vi "Debugger.vi"(8 "error in (no error)":errorcluster, 11 "Debugger In":refnum<class "Debugger.lvclass">) -> (0 "error out":errorcluster, 3 "Debugger Out":refnum<class "Debugger.lvclass">)   [LabVIEW 2020, in "Debugger.lvclass"]
uses:
  Debugger.lvclass
  Chronological List/Chronological List.lvclass
  C:/Users/anton/Documents/GitHub/triarc-debugger/source/Debug Log View/Debug Log View.lvclass
  Debugger.lvclass/Debugger.ctl
  Debug Log View/Debug Log View.lvclass
  TypeDefs/Debug Data.ctl
  <vilib>/Utility/miscctls.llb/LVPositionTypeDef.ctl
  <vilib>/Utility/miscctls.llb/LVRowAndColumnTypeDef.ctl
panel:
  in  "Processes":i32[](listbox)
  in  "Messages":i32[](listbox)
  in  "Message Log":i32(listbox)
  in  "Clear":bool
  out "Message data":variant
  in  "Received Messages":bool=TRUE
  in  "Sent Messages":bool=TRUE
  in  "Auto-Scroll":bool=TRUE
  in  "View":enum32{"Chronological", "Grouped"}(radio)
  out "Debugger enabled?":bool
  # "- Grouping"
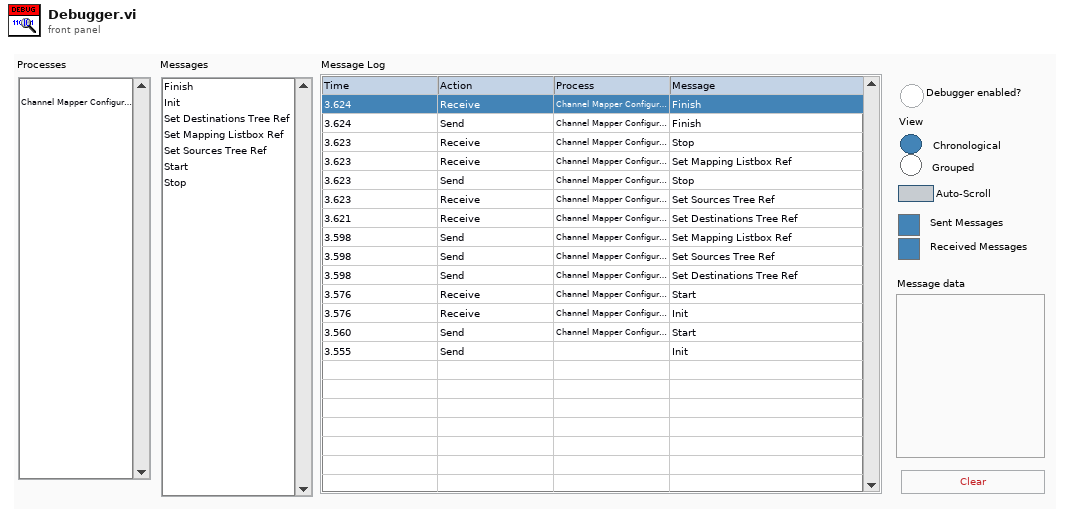
[diagram p1: front panel]
types:
  T1 = cluster{"Action":string, "Call Chain":string, "Process":string, "Message":string, "Message Data":variant, "Time":u32}
  T2 = typedef "Debugger.lvclass/Debug Data.ctl" = cluster{"Action":string, "Call Chain":string, "Process":string, "Message":string, "Message Data":variant, "Time":u32}
  T3 = typedef "LVPositionTypeDef.ctl" = cluster{"Left":i32, "Top":i32}
  T4 = typedef "LVRowAndColumnTypeDef.ctl" = cluster{"Row":i32, "Column":i32}
  T5 = typedef "LVRectTypeDef.ctl" = cluster{"Left":i16, "Top":i16, "Right":i16, "Bottom":i16}
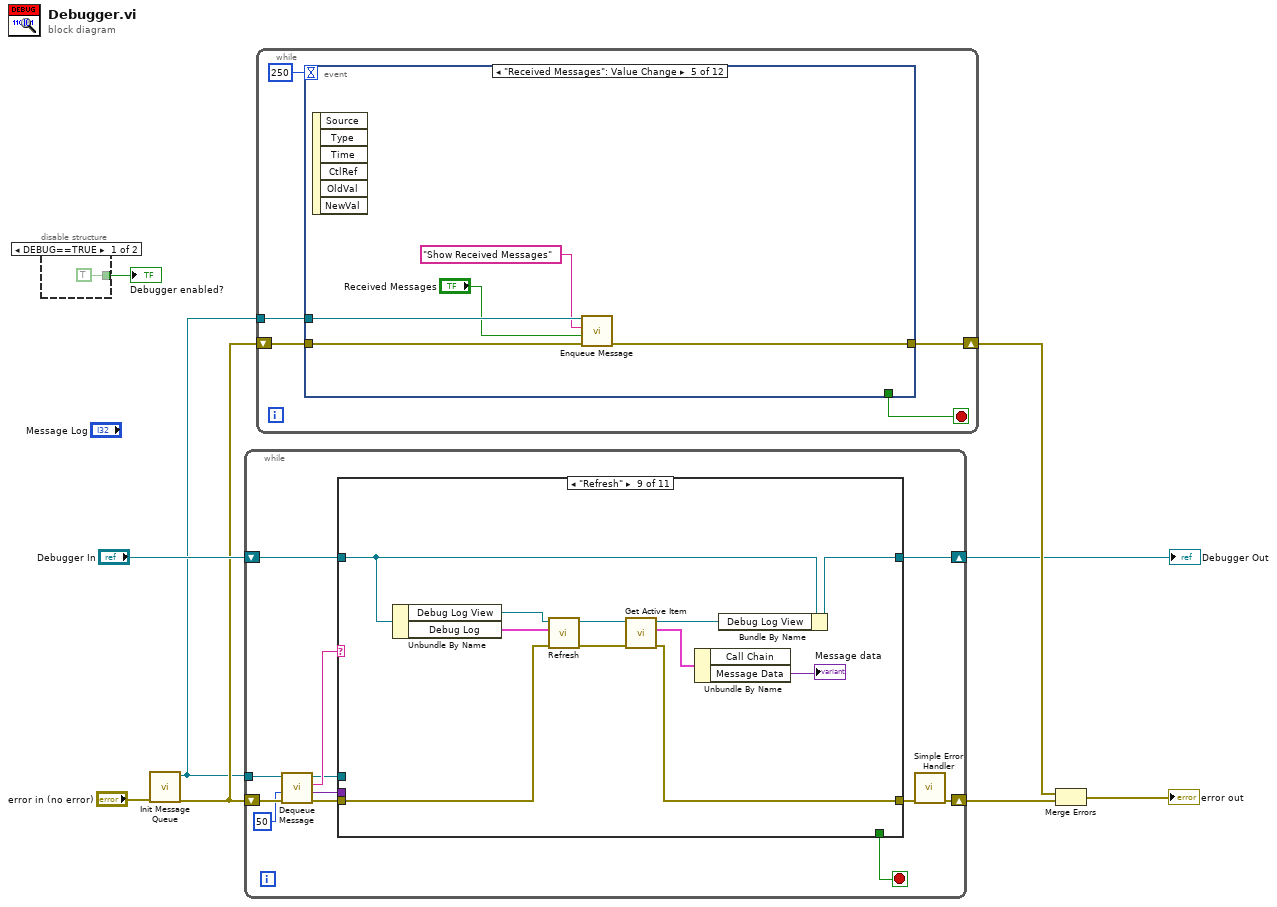
[diagram p0: block diagram]
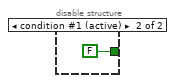
[diagram p2: hidden frame]
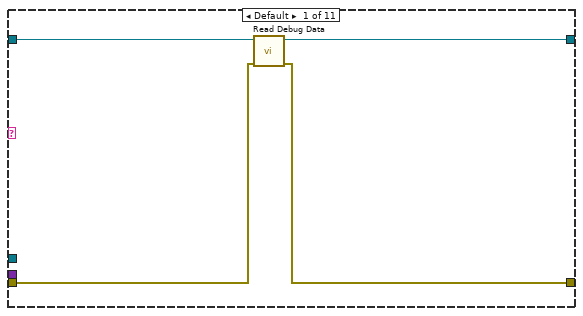
[diagram p3: hidden frame]
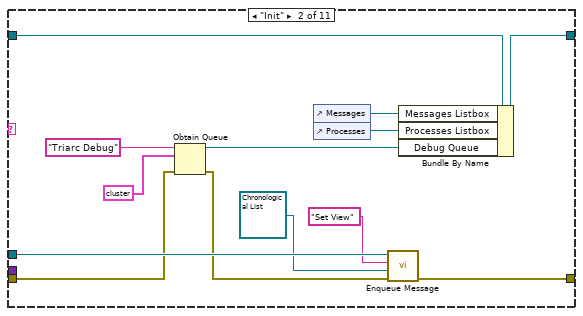
[diagram p4: hidden frame]
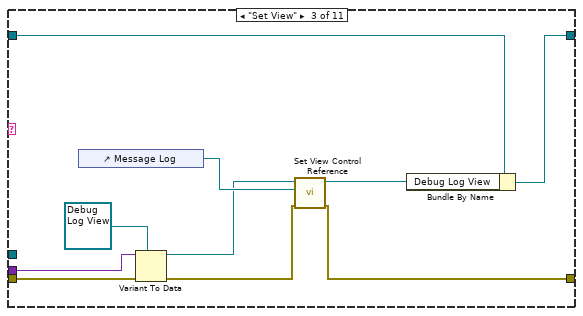
[diagram p5: hidden frame]
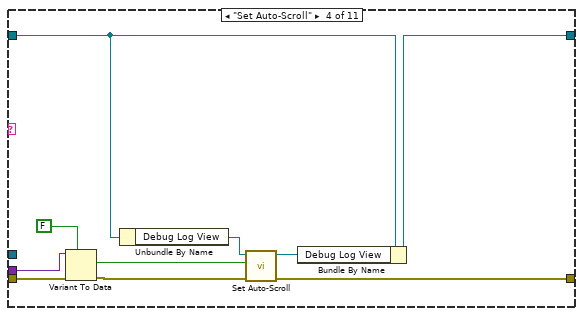
[diagram p6: hidden frame]
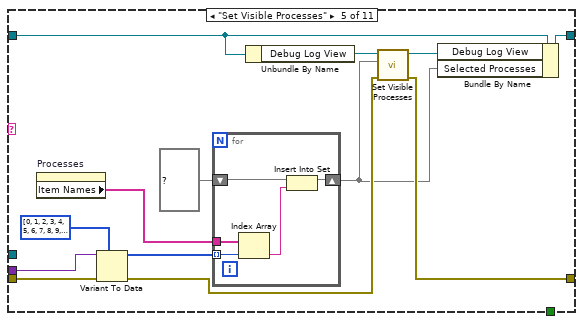
[diagram p7: hidden frame]
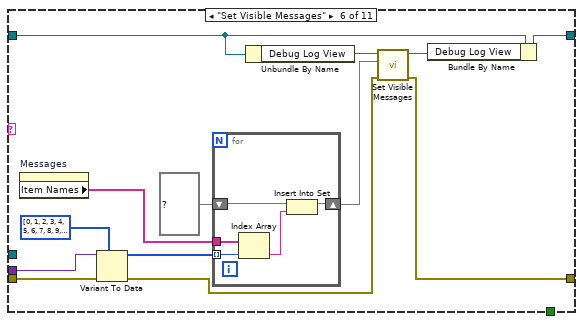
[diagram p8: hidden frame]
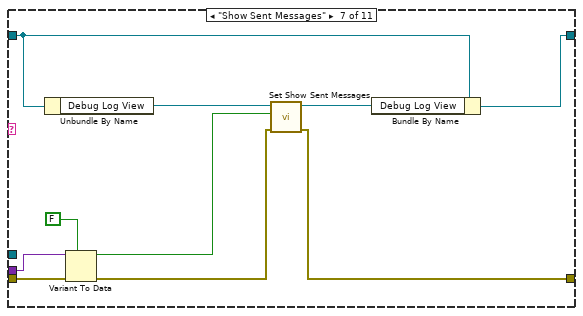
[diagram p9: hidden frame]
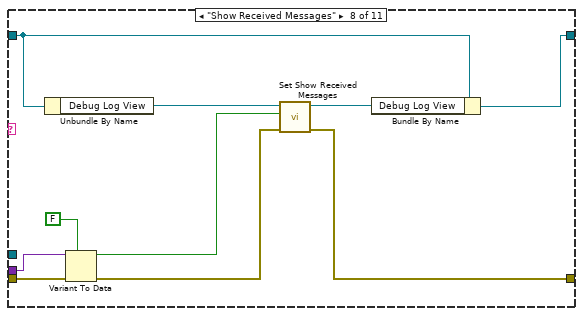
[diagram p10: hidden frame]
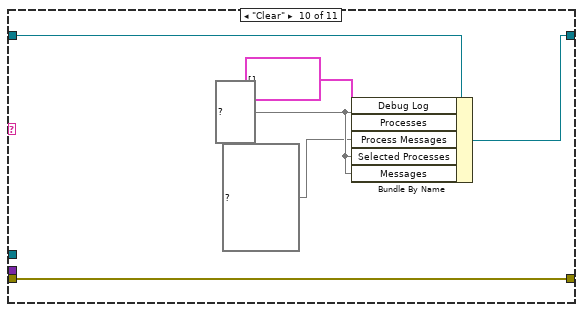
[diagram p11: hidden frame]
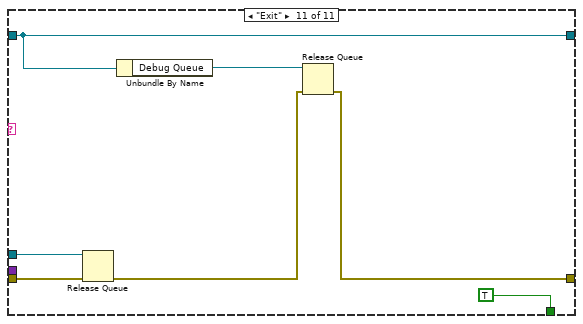
[diagram p12: hidden frame]
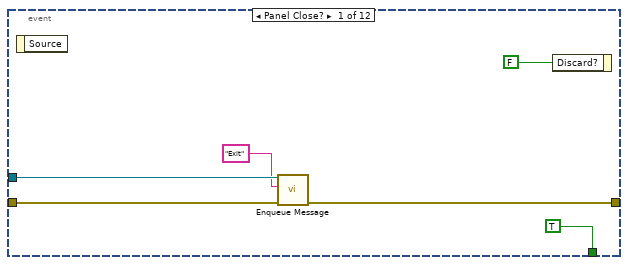
[diagram p13: hidden frame]
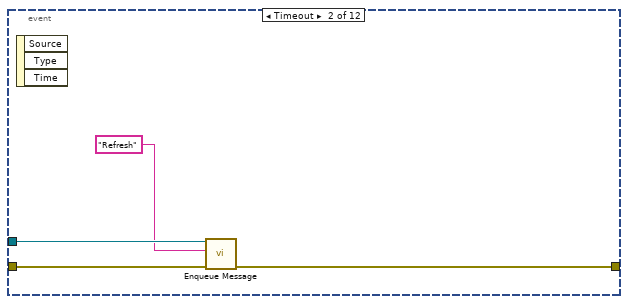
[diagram p14: hidden frame]
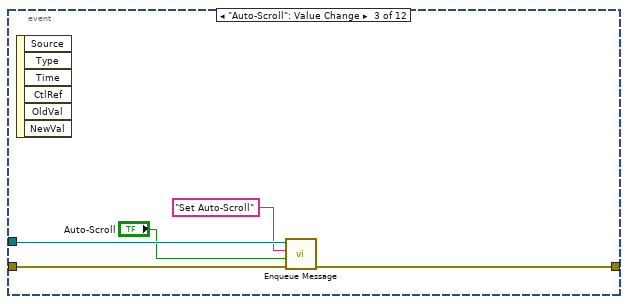
[diagram p15: hidden frame]
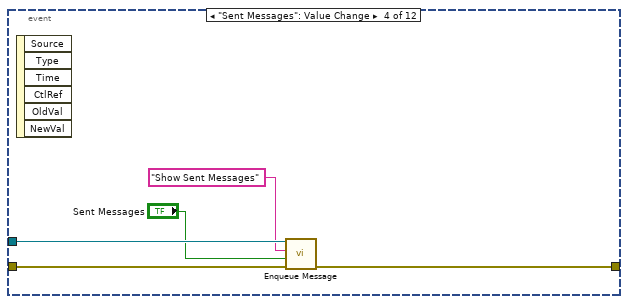
[diagram p16: hidden frame]
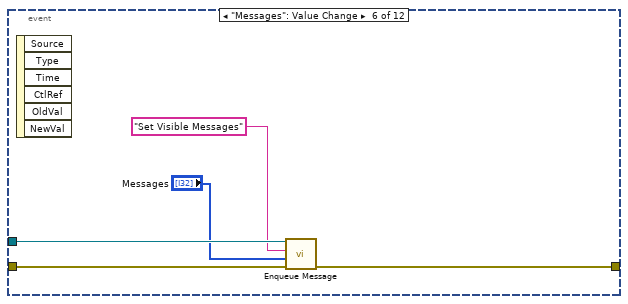
[diagram p17: hidden frame]
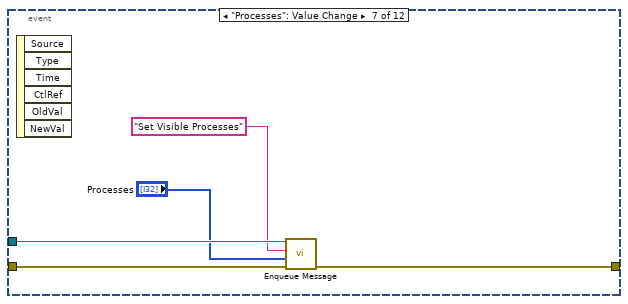
[diagram p18: hidden frame]
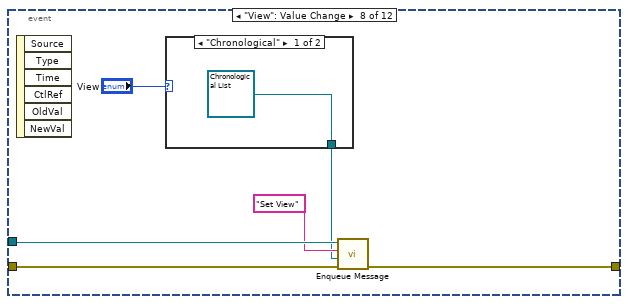
[diagram p19: hidden frame]
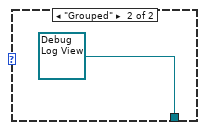
[diagram p20: hidden frame]
diagram:
  n1 = disable-structure shown="DEBUG==TRUE" {
    disable-tunnel: [TRUE FALSE ("Debugger enabled?")] -> w8
    frame condition #0 {
    }
    frame condition #1 (active) {
    }
  }
  "Debugger enabled?" <- w8
  n2 = call "Init Message Queue.vi"("error in (no error)"="error in (no error)") -> ("error out"=w5:errorcluster, "Queue out"=w4:refnum<queue>)  [unwired: 9 in]
  n3 = while {
    shift-right: [w22] -> w3
    shift-left: "Debugger In" -> [w23]
    shift-right: [w12] -> w1
    shift-left: w5 -> [w18]
    tunnel: w4 -> [w21]
    stop <- w14 stop-if-true
    n4 = call "Dequeue Message.vi"("error in (no error)"=w18, "timeout in ms (-1)"=50, "Queue in"=w21) -> ("error out"=w16:errorcluster, "Message Data"=w19:variant, "Message"=w20:string, "Queue out"=w15:refnum<queue>)  [unwired: 5 in]
    n5 = case shown="\"Refresh\"" w20 {
      tunnel: [w24 w36 w48 w52 w66 w82 w102 w112 w125 w132 w138] -> w22
      tunnel: w23 -> [w27 w40 w49 w53 w67 w83 w103 w113 w127 w133 w138]
      tunnel: w19 -> [_ _ w43 w59 w73 w91 w105 w115 _ _ _]
      tunnel: [w25 w32 w46 w55 w64 w80 w97 w107 w119 w131 w137] -> w17
      tunnel: w16 -> [w26 w34 w45 w60 w72 w90 w106 w116 w126 w131 w135]
      tunnel: w15 -> [_ w39 _ _ _ _ _ _ _ _ w136]
      tunnel: [_ _ _ _ _ _ _ _ _ _ TRUE] -> w14
      frame Default {
        n6 = call "Read Debug Data.vi"("error in (no error)"=w26, "Debugger in"=w27) -> ("error out"=w25:errorcluster, "Debugger out"=w24:refnum<class "Debugger.lvclass">)  [unwired: 8 in]
      }
      frame "Init" {
        n7 = Obtain Queue(name (unnamed)="Triarc Debug", element data type=T1 {"Action"="", "Call Chain"="", "Process"="", "Message"="", "Message Data"=variant, "Time"=0} ("output cluster"), error in (no error)=w34) -> (queue out=w35:refnum<queue>, error out=w33:errorcluster)  [unwired: 2 in, 1 out]
        n8 = control-ref of="Messages"() -> (w28:refnum<vi>)
        n9 = control-ref of="Processes"() -> (w29:refnum<vi>)
        n10 = call "Enqueue Message.vi"("error in (no error)"=w33, "Message Data"=refnum<class "Chronological List.lvclass"> refnum ("Debugger.lvlib:Chronological List.lvclass"), "Message"="Set View", "Queue in"=w39) -> ("error out"=w32:errorcluster)  [unwired: 6 in, 1 out]
        n11 = Bundle By Name(cluster=w40, "Messages Listbox"=w28, "Processes Listbox"=w29, "Debug Queue"=w35) -> (w36:refnum<class "Debugger.lvclass">)
      }
      frame "Set View" {
        n12 = control-ref of="Message Log"() -> (w50:refnum<vi>)
        n13 = Variant To Data(error in=w45, type=refnum<class "Debug Log View.lvclass"> refnum ("Debug Log View"), Variant=w43) -> (data=w41:refnum<class "Debug Log View.lvclass">, error out=w44:errorcluster)
        n14 = call-dynamic "Set View Control Reference.vi"("error in (no error)"=w44, "View Control"=w50, "Debug Log View in"=w41) -> ("error out"=w46:errorcluster, "Debug Log View out"=w47:refnum<class "Debug Log View.lvclass">)  [unwired: 7 in]
        n15 = Bundle By Name(cluster=w49, "Debug Log View"=w47) -> (w48:refnum<class "Debugger.lvclass">)
      }
      frame "Set Auto-Scroll" {
        n16 = Variant To Data(error in=w60, type=FALSE, Variant=w59) -> (data=w57:bool, error out=w56:errorcluster)
        n17 = Unbundle By Name(w53) -> ("Debug Log View"=w54:refnum<class "Debug Log View.lvclass">)
        n18 = call-dynamic "Set Auto-Scroll.vi"("error in (no error)"=w56, "Auto-Scroll?"=w57, "Debug Log View in"=w54) -> ("error out"=w55:errorcluster, "Debug Log View out"=w51:refnum<class "Debug Log View.lvclass">)  [unwired: 7 in]
        n19 = Bundle By Name(cluster=w53, "Debug Log View"=w51) -> (w52:refnum<class "Debugger.lvclass">)
      }
      frame "Set Visible Processes" {
        n20 = property on="Processes" class="LstBox (strict)"() -> ("Item Names"=w62:string[])  [unwired: 2 in, 2 out]
        n21 = Variant To Data(error in=w72, type=i32[] [0, 1, 2, 3, 4, 5, 6, 7, 8, 9, 10, 11, 12, 13, 14, 15, 16, 17, 18, 19, 20, 21, 22] ("Message Filter"), Variant=w73) -> (data=w70:i32[], error out=w63:errorcluster)
        n22 = for {
          tunnel: w62 -> [w78]
          tunnel: w70 -> [w77] mode=indexing
          shift-right: [w74] -> w61
          shift-left: set{string} {} ("set in") -> [w76]
          n23 = Index Array(array=w78, index=w77) -> (element=w75:string)
          n24 = Insert Into Set(10:w75, 11:w76) -> (3:w74:set{string})  [unwired: 1 out]
        }
        n25 = Unbundle By Name(w67) -> ("Debug Log View"=w68:refnum<class "Debug Log View.lvclass">)
        n26 = call-dynamic "Set Visible Processes.vi"("error in (no error)"=w63, "Processes"=w61, "Debug Log View In"=w68) -> ("error out"=w64:errorcluster, "Debug Log View Out"=w65:refnum<class "Debug Log View.lvclass">)  [unwired: 7 in]
        n27 = Bundle By Name(cluster=w67, "Debug Log View"=w65, "Selected Processes"=w61) -> (w66:refnum<class "Debugger.lvclass">)
      }
      frame "Set Visible Messages" {
        n28 = property on="Messages" class="LstBox (strict)"() -> ("Item Names"=w88:string[])  [unwired: 2 in, 2 out]
        n29 = Variant To Data(error in=w90, type=i32[] [0, 1, 2, 3, 4, 5, 6, 7, 8, 9, 10, 11, 12, 13, 14, 15, 16, 17, 18, 19, 20, 21, 22] ("Message Filter"), Variant=w91) -> (data=w87:i32[], error out=w79:errorcluster)
        n30 = for {
          tunnel: w88 -> [w96]
          tunnel: w87 -> [w95] mode=indexing
          shift-right: [w92] -> w85
          shift-left: set{string} {} ("set in") -> [w94]
          n31 = Index Array(array=w96, index=w95) -> (element=w93:string)
          n32 = Insert Into Set(10:w93, 11:w94) -> (3:w92:set{string})  [unwired: 1 out]
        }
        n33 = Unbundle By Name(w83) -> ("Debug Log View"=w84:refnum<class "Debug Log View.lvclass">)
        n34 = call-dynamic "Set Visible Messages.vi"("error in (no error)"=w79, "Messages"=w85, "Debug Log View in"=w84) -> ("error out"=w80:errorcluster, "Debug Log View out"=w81:refnum<class "Debug Log View.lvclass">)  [unwired: 7 in]
        n35 = Bundle By Name(cluster=w83, "Debug Log View"=w81) -> (w82:refnum<class "Debugger.lvclass">)
      }
      frame "Show Sent Messages" {
        n36 = Unbundle By Name(w103) -> ("Debug Log View"=w99:refnum<class "Debug Log View.lvclass">)
        n37 = Variant To Data(error in=w106, type=FALSE, Variant=w105) -> (data=w100:bool, error out=w101:errorcluster)
        n38 = call-dynamic "Set Show Sent Messages.vi"("error in (no error)"=w101, "Show Sent Messages?"=w100, "Debug Log View In"=w99) -> ("error out"=w97:errorcluster, "Debug Log View Out"=w98:refnum<class "Debug Log View.lvclass">)  [unwired: 7 in]
        n39 = Bundle By Name(cluster=w103, "Debug Log View"=w98) -> (w102:refnum<class "Debugger.lvclass">)
      }
      frame "Show Received Messages" {
        n40 = Unbundle By Name(w113) -> ("Debug Log View"=w109:refnum<class "Debug Log View.lvclass">)
        n41 = Variant To Data(error in=w116, type=FALSE, Variant=w115) -> (data=w110:bool, error out=w111:errorcluster)
        n42 = call-dynamic "Set Show Received Messages.vi"("error in (no error)"=w111, "Show Received Messages?"=w110, "Debug Log View In"=w109) -> ("error out"=w107:errorcluster, "Debug Log View Out"=w108:refnum<class "Debug Log View.lvclass">)  [unwired: 7 in]
        n43 = Bundle By Name(cluster=w113, "Debug Log View"=w108) -> (w112:refnum<class "Debugger.lvclass">)
      }
      frame "Refresh" {
        n44 = Unbundle By Name(w127) -> ("Debug Log View"=w124:refnum<class "Debug Log View.lvclass">, "Debug Log"=w123:T2[])
        n45 = call-dynamic "Refresh.vi"("error in (no error)"=w126, "Debug Log"=w123, "Debug Log View In"=w124) -> ("error out"=w120:errorcluster, "Debug Log View Out"=w122:refnum<class "Debug Log View.lvclass">)  [unwired: 7 in]
        n46 = call-dynamic "Get Active Item.vi"("error in (no error)"=w120, "Debug Log View In"=w122) -> ("error out"=w119:errorcluster, "Debug Data"=w118:T2, "Debug Log View Out"=w121:refnum<class "Debug Log View.lvclass">)  [unwired: 7 in]
        n47 = Unbundle By Name(w118) -> ("Message Data"=→"Message data":variant)  [unwired: 1 out]
        n48 = Bundle By Name(cluster=w127, "Debug Log View"=w121) -> (w125:refnum<class "Debugger.lvclass">)
      }
      frame "Clear" {
        w129 = set{string} {} ("Processes")
        n49 = Bundle By Name(cluster=w133, "Debug Log"=T2[] [], "Processes"=w129, "Process Messages"=map{string, set{string}} {}, "Selected Processes"=w129, "Messages"=w129) -> (w132:refnum<class "Debugger.lvclass">)
      }
      frame "Exit" {
        n50 = Release Queue(queue=w136, error in (no error)=w135) -> (error out=w134:errorcluster)  [unwired: 1 in, 2 out]
        n51 = Unbundle By Name(w138) -> ("Debug Queue"=w139:refnum<queue>)
        n52 = Release Queue(queue=w139, error in (no error)=w134) -> (error out=w137:errorcluster)  [unwired: 1 in, 2 out]
      }
    }
    n53 = call <vilib>:"Simple Error Handler.vi"("error in (no error)"=w17) -> ("error out"=w12:errorcluster)  [unwired: 4 in, 4 out]
  }
  "Debugger Out" <- w3
  n54 = while {
    shift-right: [w145] -> w9
    shift-left: w5 -> [w144]
    tunnel: w4 -> [w141]
    stop <- w143 stop-if-true
    n55 = event shown="[4] \"Received Messages\": Value Change" {
      selector: _ -> [_ _ _ _ _ _ _ _ _ _ _ _]
      dyn-events: _ -> [_ _ _ _ _ _ _ _ _ _ _ _]
      timeout: 250 -> [_ _ _ _ _ _ _ _ _ _ _ _]
      tunnel: [w148 w154 w159 w164 w169 w174 w179 w185 w190 w192 w199 w213] -> w145
      tunnel: w144 -> [w151 w155 w160 w165 w170 w175 w180 w186 w190 w192 w199 w214]
      tunnel: [TRUE _ _ _ _ _ _ _ _ _ _ _] -> w143
      tunnel: w141 -> [w147 w153 w158 w163 w168 w173 w178 w184 _ _ _ w212]
      event Panel Close? {
        n56 = event-data() -> ()  [unwired: 1 in, 1 out]
        n57 = call "Enqueue Message.vi"("error in (no error)"=w151, "Message"="Exit", "Queue in"=w147) -> ("error out"=w148:errorcluster)  [unwired: 7 in, 1 out]
        n58 = event-data("Discard?"=FALSE) -> ()  [unwired: 1 in, 1 out]
      }
      event Timeout {
        n59 = event-data() -> ()  [unwired: 1 in, 3 out]
        n60 = call "Enqueue Message.vi"("error in (no error)"=w155, "Message"="Refresh", "Queue in"=w153) -> ("error out"=w154:errorcluster)  [unwired: 7 in, 1 out]
      }
      event "Auto-Scroll": Value Change {
        n61 = event-data() -> ()  [unwired: 1 in, 6 out]
        n62 = call "Enqueue Message.vi"("error in (no error)"=w160, "Message Data"="Auto-Scroll", "Message"="Set Auto-Scroll", "Queue in"=w158) -> ("error out"=w159:errorcluster)  [unwired: 6 in, 1 out]
      }
      event "Sent Messages": Value Change {
        n63 = event-data() -> ()  [unwired: 1 in, 6 out]
        n64 = call "Enqueue Message.vi"("error in (no error)"=w165, "Message Data"="Sent Messages", "Message"="Show Sent Messages", "Queue in"=w163) -> ("error out"=w164:errorcluster)  [unwired: 6 in, 1 out]
      }
      event "Received Messages": Value Change {
        n65 = event-data() -> ()  [unwired: 1 in, 6 out]
        n66 = call "Enqueue Message.vi"("error in (no error)"=w170, "Message Data"="Received Messages", "Message"="Show Received Messages", "Queue in"=w168) -> ("error out"=w169:errorcluster)  [unwired: 6 in, 1 out]
      }
      event "Messages": Value Change {
        n67 = event-data() -> ()  [unwired: 1 in, 6 out]
        n68 = call "Enqueue Message.vi"("error in (no error)"=w175, "Message Data"="Messages", "Message"="Set Visible Messages", "Queue in"=w173) -> ("error out"=w174:errorcluster)  [unwired: 6 in, 1 out]
      }
      event "Processes": Value Change {
        n69 = event-data() -> ()  [unwired: 1 in, 6 out]
        n70 = call "Enqueue Message.vi"("error in (no error)"=w180, "Message Data"="Processes", "Message"="Set Visible Processes", "Queue in"=w178) -> ("error out"=w179:errorcluster)  [unwired: 6 in, 1 out]
      }
      event "View": Value Change {
        n71 = event-data() -> ()  [unwired: 1 in, 6 out]
        n72 = case shown="\"Chronological\"" "View" {
          tunnel: [refnum<class "Chronological List.lvclass"> refnum ("Debugger.lvlib:Chronological List.lvclass") refnum<class "Debug Log View.lvclass"> refnum ("Debugger.lvlib:Debug Log View.lvclass")] -> w181
          frame "Chronological" {
          }
          frame "Grouped" {
          }
        }
        n73 = call "Enqueue Message.vi"("error in (no error)"=w186, "Message Data"=w181, "Message"="Set View", "Queue in"=w184) -> ("error out"=w185:errorcluster)  [unwired: 6 in, 1 out]
      }
      event Pane Size {
        n74 = event-data() -> ()  [unwired: 1 in, 1 out]
        n75 = property on="Processes" class="LstBox (strict)"("Position"=T3 {"Left"=2, "Top"=2}) -> ()  [unwired: 2 in, 2 out]
      }
      event Pane Size {
        n76 = event-data() -> ()  [unwired: 1 in, 6 out]
        n77 = property on="Messages" class="LstBox (strict)"("Position"=T3 {"Left"=2, "Top"=2}) -> ()  [unwired: 2 in, 2 out]
      }
      event Pane Size {
        n78 = event-data() -> ("NewBnds"=w197:T5)  [unwired: 1 in, 5 out]
        n79 = Unbundle By Name(w197) -> ("Right"=w196:i16, "Left"=w195:i16)
        n80 = Subtract(x=w196, y=w195) -> (x-y=w193:i16)
        n81 = for {
          N: 4 -> [_]
          tunnel: w193 -> [w202]
          i -> [w203]
          n82 = Bundle By Name(cluster=T4 {"Row"=0, "Column"=0} ("Active Cell:Active Cell"), "Column"=w203) -> (w204:T4)
          n83 = case shown="Default" w203 {
            tunnel: [0.0 0.2 0.2 0.2 0.4] -> w200
            frame Default {
            }
            frame 0 {
            }
            frame 1 {
            }
            frame 2 {
            }
            frame 3 {
            }
          }
          n84 = Multiply(x=w202, y=w200) -> (x*y=w201:dbl)
          n85 = property on="Message Log" class="MCListbox (strict)"("ActiveCell"=w204, "Width"=w201) -> ()  [unwired: 2 in, 2 out]
        }
        n86 = property on="Message Log" class="MCListbox (strict)"("Position"=T3 {"Left"=2, "Top"=2}) -> ()  [unwired: 2 in, 2 out]
      }
      event "Clear": Value Change {
        n87 = event-data() -> ()  [unwired: 1 in, 6 out]
        n88 = call "Enqueue Message.vi"("error in (no error)"=w214, "Message"="Clear", "Queue in"=w212) -> ("error out"=w213:errorcluster)  [unwired: 7 in, 1 out]
      }
    }
  }
  n89 = Merge Errors(w9, w1) -> (→"error out":errorcluster)
